vi "hmi_progress.vi"(7 "hmi_references":T1, 8 "error in (no error)":errorcluster, 10 "current_index":i32, 11 "total_operations":i32) -> (0 "error out":errorcluster)   [LabVIEW 2015, in "lv-build-interface.lvlib"]
uses:
  lv-build-interface.lvlib
  _controls/hmi_references.ctl
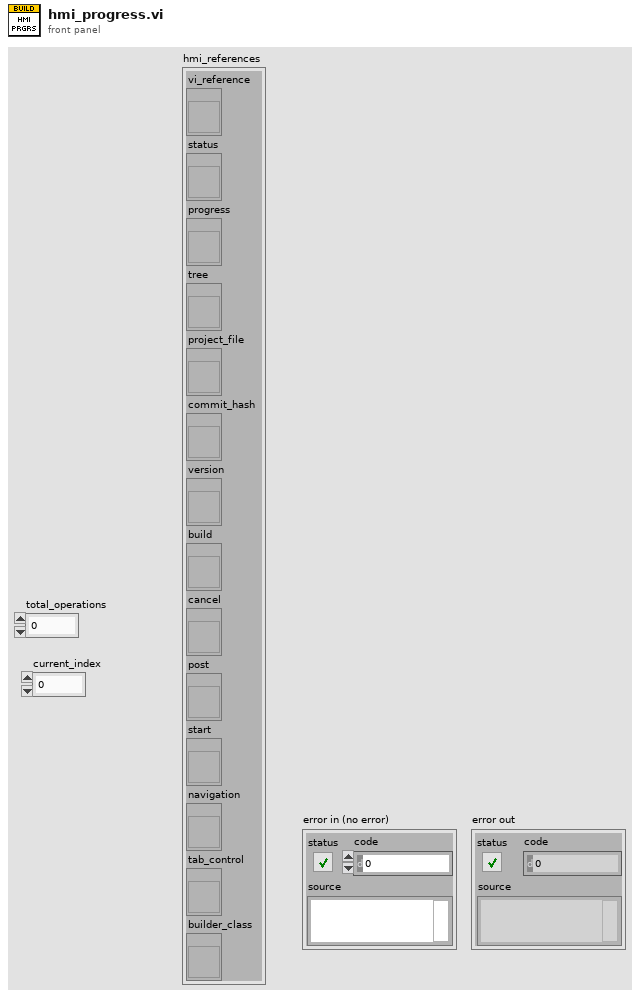
[diagram p1: front panel]
types:
  T1 = typedef "lv-build-interface.lvlib/hmi_references.ctl" = cluster{"vi_reference":refnum<vi>, "status":refnum<vi>, "progress":refnum<vi>, "tree":refnum<vi>, "project_file":refnum<vi>, "commit_hash":refnum<vi>, "version":refnum<vi>, "build":refnum<vi>, "cancel":refnum<vi>, "post":refnum<vi>, "start":refnum<vi>, "navigation":refnum<vi>, "tab_control":refnum<vi>, "builder_class":refnum<vi>}
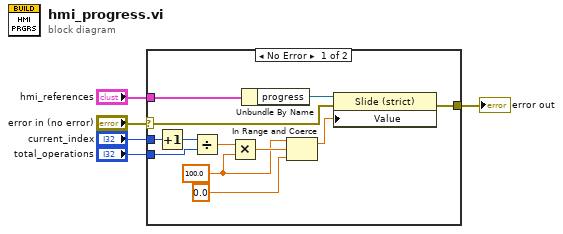
[diagram p0: block diagram]
diagram:
  n1 = case shown="No Error" "error in (no error)" {
    selector: "error in (no error)" -> [w15 w18]
    tunnel: "hmi_references" -> [w17 _]
    tunnel: "total_operations" -> [w13 _]
    tunnel: [w14 w18] -> w2
    tunnel: "current_index" -> [w12 _]
    frame No Error {
      w8 = 100.0 ("x")
      n2 = Increment(x=w12) -> (x+1=w6:i32)
      n3 = Divide(x=w6, y=w13) -> (x/y=w11:dbl)
      n4 = Multiply(x=w11, y=w8) -> (x*y=w10:dbl)
      n5 = Unbundle By Name(w17) -> ("progress"=w16:refnum<vi>)
      n6 = In Range and Coerce(upper limit=w8, x=w10, lower limit=0.0) -> (coerced(x)=w9:dbl)  [unwired: 1 out]
      n7 = property class="Slide (strict)"(reference=w16, error in=w15, "Value"=w9) -> (error out=w14:errorcluster)  [unwired: 1 out]
    }
    frame Error {
    }
  }
  "error out" <- w2
